vi "ReadDAQConfig.vi"(8 "error in":errorcluster caption="错误输入（无错误）", 11 "产品型号":refnum<vi>) -> (0 "error out":errorcluster caption="错误输出", 3 "DAQConfig":T1={"DIO"=[["ACC", "Dev1/port2/line0", "Dev1/port0/line24"], ["ILL", "Dev1/port2/line1", "Dev1/port0/line25"], ["BACK", "Dev1/port2/line2", "Dev1/port0/line26"], ["BRAKE", "Dev1/port2/line3", "Dev1/port0/line27"], ["PowerON_Vps", "Dev1/port2/line4", "Dev1/port0/line28"], ["PowerON_+B", "Dev1/port2/line5", "Dev1/port0/line29"], ["SW", "Dev1/port2/line6", "Dev1/port0/line30"], ["SW1", "Dev1/port0/line5", "Dev1/port0/line13"], ["SW2", "Dev1/port0/line6", "Dev1/port0/line14"], ["LineOut1", "Dev1/port1/line3", "Dev1/port0/line19"], ["LineOut2", "Dev1/port1/line2", "Dev1/port0/line18"], ["LineOut3", "Dev1/port1/line5", "Dev1/port0/line21"], ["LineOut4", "Dev1/port1/line4", "Dev1/port0/line20"], ["LineOut5", "Dev1/port1/line7", "Dev1/port0/line23"], ["LineOut6", "Dev1/port1/line6", "Dev1/port0/line22"], ["SPK", "Dev1/port2/line7", "Dev1/port0/line31"], ["SPK2", "Dev1/port0/line7", "Dev1/port0/line15"], ["IPOD_DET", "Dev1/port1/line0", "Dev1/port0/line16"], ["RING", "Dev1/port1/line1", "Dev1/port0/line17"], ["PASSButton", "Dev1/port0/line2", "Dev1/port0/line10"], ["FAILButton", "Dev1/port0/line3", "Dev1/port0/line11"], ["DO_IPOD+5V", "Dev1/port0/line4", "Dev1/port0/line12"]], "AO"=[["PowerSimulate", "Dev1/ao0", "Dev1/ao2"], ["AudioSW", "Dev1/ao1", "Dev1/ao3"]], "AI"=[["PowerMonitor", "Dev1/ai5", "Dev1/ai21"], ["FL", "Dev1/ai0", "Dev1/ai16"], ["FR", "Dev1/ai1", "Dev1/ai17"], ["RL", "Dev1/ai2", "Dev1/ai18"], ["RR", "Dev1/ai3", "Dev1/ai19"], ["FLOUT", "Dev1/ai6", "Dev1/ai22"], ["FROUT", "Dev1/ai7", "Dev1/ai23"], ["RLOUT", "Dev1/ai13", "Dev1/ai29"], ["RROUT", "Dev1/ai14", "Dev1/ai30"], ["SUB", "Dev1/ai15", "Dev1/ai31"], ["Current", "Dev1/ai4", "Dev1/ai20"], ["IPOD+5V", "Dev1/ai12", "Dev1/ai28"]]})   [LabVIEW 2013]
uses:
  Controls/DAQConfig.ctl
  <vilib>/Utility/NIReport.llb/NI_report.lvclass
  GlobalValue.vi
  <vilib>/addons/_office/excel.llb/Excel Get Data ([str]).vi
  <vilib>/addons/_office/NI_ReportGenerationToolkit.lvlib
  <vilib>/Utility/NIReport.llb/Excel/NI_Excel.lvclass
panel:
  out "AI":string[][](table)=[["PowerMonitor", "Dev1/ai5", "Dev1/ai21"], ["FL", "Dev1/ai0", "Dev1/ai16"], ["FR", "Dev1/ai1", "Dev1/ai17"], ["RL", "Dev1/ai2", "Dev1/ai18"], ["RR", "Dev1/ai3", "Dev1/ai19"], ["FLOUT", "Dev1/ai6", "Dev1/ai22"], ["FROUT", "Dev1/ai7", "Dev1/ai23"], ["RLOUT", "Dev1/ai13", "Dev1/ai29"], ["RROUT", "Dev1/ai14", "Dev1/ai30"], ["SUB", "Dev1/ai15", "Dev1/ai31"], ["Current", "Dev1/ai4", "Dev1/ai20"], ["IPOD+5V", "Dev1/ai12", "Dev1/ai28"]]
  out "AO":string[][](table)=[["PowerSimulate", "Dev1/ao0", "Dev1/ao2"], ["AudioSW", "Dev1/ao1", "Dev1/ao3"]]
  out "DO":string[][](table)=[["ACC", "Dev1/port2/line0", "Dev1/port0/line24"], ["ILL", "Dev1/port2/line1", "Dev1/port0/line25"], ["BACK", "Dev1/port2/line2", "Dev1/port0/line26"], ["BRAKE", "Dev1/port2/line3", "Dev1/port0/line27"], ["PowerON_Vps", "Dev1/port2/line4", "Dev1/port0/line28"], ["PowerON_+B", "Dev1/port2/line5", "Dev1/port0/line29"], ["SW", "Dev1/port2/line6", "Dev1/port0/line30"], ["SW1", "Dev1/port0/line5", "Dev1/port0/line13"], ["SW2", "Dev1/port0/line6", "Dev1/port0/line14"], ["LineOut1", "Dev1/port1/line3", "Dev1/port0/line19"], ["LineOut2", "Dev1/port1/line2", "Dev1/port0/line18"], ["LineOut3", "Dev1/port1/line5", "Dev1/port0/line21"], ["LineOut4", "Dev1/port1/line4", "Dev1/port0/line20"], ["LineOut5", "Dev1/port1/line7", "Dev1/port0/line23"], ["LineOut6", "Dev1/port1/line6", "Dev1/port0/line22"], ["SPK", "Dev1/port2/line7", "Dev1/port0/line31"], ["SPK2", "Dev1/port0/line7", "Dev1/port0/line15"], ["IPOD_DET", "Dev1/port1/line0", "Dev1/port0/line16"], ["RING", "Dev1/port1/line1", "Dev1/port0/line17"], ["PASSButton", "Dev1/port0/line2", "Dev1/port0/line10"], ["FAILButton", "Dev1/port0/line3", "Dev1/port0/line11"], ["DO_IPOD+5V", "Dev1/port0/line4", "Dev1/port0/line12"]]
  out "ConfigPath":string="D:\\导航\\AVN\\config\\DAQConfig.xls"
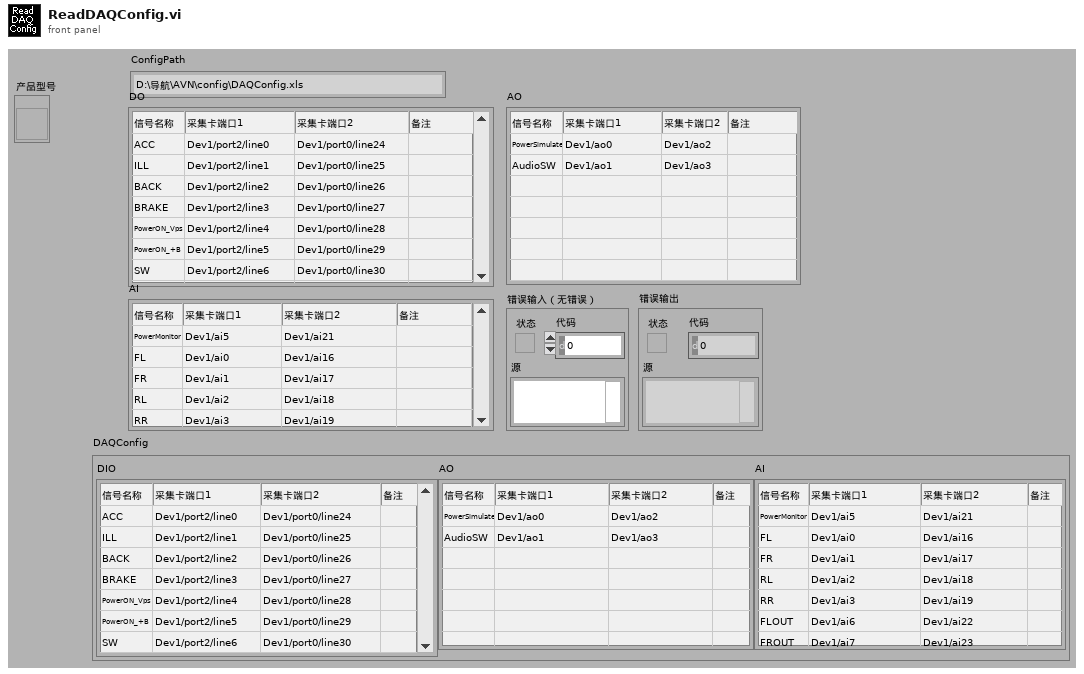
[diagram p1: front panel]
types:
  T1 = typedef "DAQConfig.ctl" = cluster{"DIO":string[][], "AO":string[][], "AI":string[][]}
  T2 = enum16{"maximized", "minimized", "normal", "no change"}
  T3 = enum16{"Standard Report", "HTML", "Word", "Excel"}
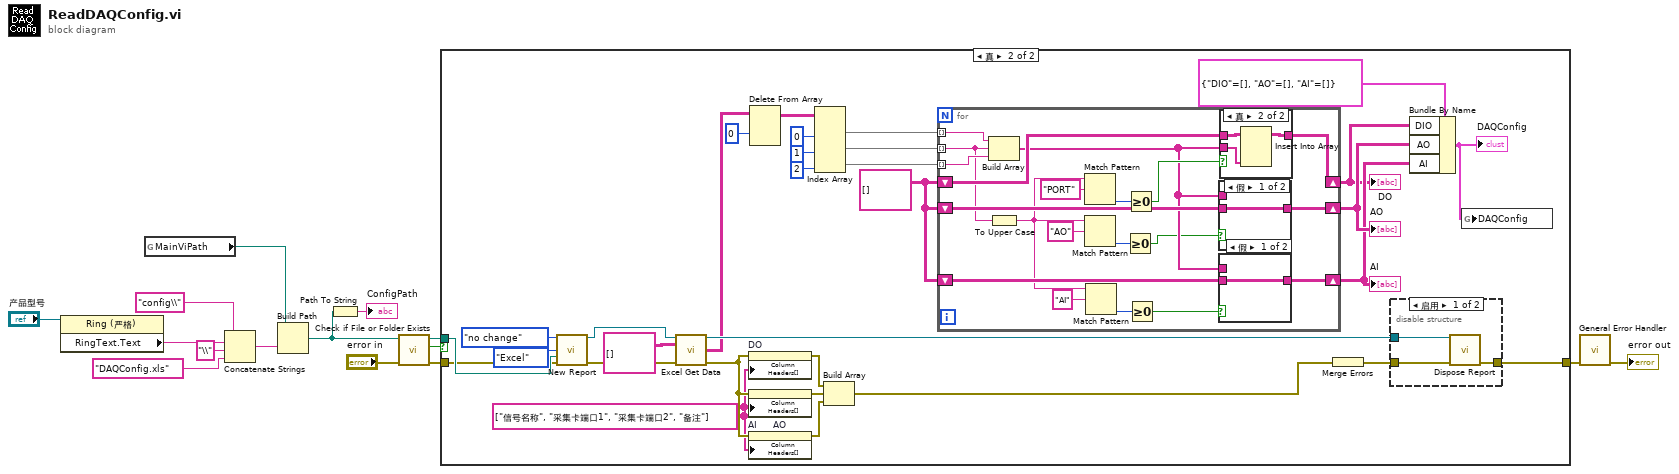
[diagram p0: block diagram]
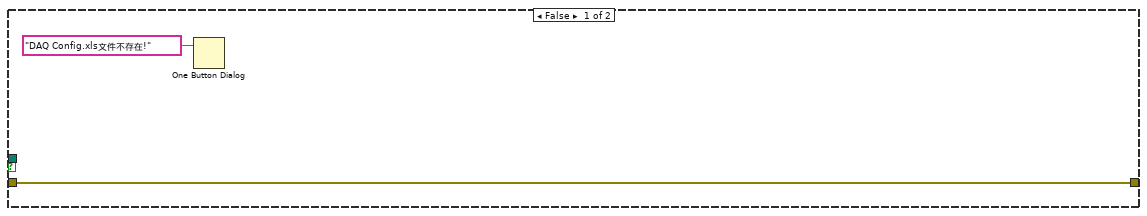
[diagram p2: hidden frame]
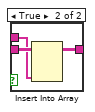
[diagram p4: hidden frame]
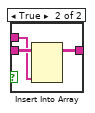
[diagram p6: hidden frame]
diagram:
  n1 = property on="属性节点" class="Ring (严格)"(reference="产品型号") -> ("RingText.Text"=w3:string)  [unwired: 1 in, 2 out]
  n2 = global read "GlobalValue.vi" "MainViPath"() -> (w7:path)
  n3 = Concatenate Strings("config\\" ("连接的字符串"), w3, "\\" ("字符串"), "DAQConfig.xls" ("连接的字符串")) -> (w1:string)
  n4 = Build Path(base path=w7, name or relative path=w1) -> (appended path=w12:path)
  n5 = Path To String(path=w12) -> (string=→"ConfigPath":string)
  n6 = call <vilib>:"Check if File or Folder Exists.vi"("error in (no error)"="error in", "path"=w12) -> ("error out"=w15:errorcluster, "file or folder exists?"=w14:bool, "dup path"=w9:path)  [unwired: 7 out]
  n7 = case shown="真" w14 {
    tunnel: w15 -> [w17 w47]
    tunnel: w9 -> [_ w48]
    tunnel: [w17 w45] -> w13
    frame False {
      n8 = One Button Dialog(message="DAQ Config.xls文件不存在!" ("消息")) -> ()  [unwired: 1 in, 1 out]
    }
    frame True {
      w26 = string[] ["信号名称", "采集卡端口1", "采集卡端口2", "备注"] ("已删除的部分")
      w24 = string[][] [] ("Array")
      n9 = call <vilib>:"New Report.vi"("window state (normal)"=T2."no change", "report type"=T3."Excel", "template (empty)"=w48, "error in (no error)"=w47) -> ("report out"=w40:refnum<class "NI_report.lvclass">, "error out"=w38:errorcluster)  [unwired: 2 in, 8 out]
      n10 = call-poly <vilib>:"Excel Get Data.vi"("report in"=w40, "data type"=string[][] [], "error in (no error)"=w38) -> ("report out"=w46:refnum<class "NI_report.lvclass">, "data"=w37:string[][], "error out"=w27:errorcluster)  [unwired: 10 in]
      n11 = property on="DO" class="Tbl (严格)"(error in=w27, "Column Headers[]"=w26) -> (error out=w22:errorcluster)  [unwired: 1 in, 1 out]
      n12 = property on="AO" class="Tbl (严格)"(error in=w27, "Column Headers[]"=w26) -> (error out=w39:errorcluster)  [unwired: 1 in, 1 out]
      n13 = property on="AI" class="Tbl (严格)"(error in=w27, "Column Headers[]"=w26) -> (error out=w25:errorcluster)  [unwired: 1 in, 1 out]
      n14 = Delete From Array(array=w37, index (row)=0 ("索引 (行)")) -> (array with subset deleted=w35:string[][])  [unwired: 2 in, 1 out]
      n15 = Index Array(array=w35, index (col) #1=0 ("禁用的索引 (列)"), index (col) #2=1 ("索引 (列)"), index (col) #3=2 ("索引 (列)")) -> (element #1=w33:string[], element #2=w21:string[], element #3=w19:string[])  [unwired: 3 in]
      n16 = Build Array(w22, w39, w25) -> (w43:errorcluster[])
      n17 = for {
        shift-right: [w66] -> w23
        shift-left: w24 -> [w65]
        shift-right: [w70] -> w29
        shift-left: w24 -> [w69]
        tunnel: w33 -> [w58] mode=indexing
        shift-right: [w62] -> w28
        shift-left: w24 -> [w63]
        tunnel: w21 -> [w57] mode=indexing
        tunnel: w19 -> [w61] mode=indexing
        n18 = Build Array(w58, w57, w61) -> (w59:string[])
        n19 = To Upper Case(1:w57) -> (0:w60:string)
        n20 = Match Pattern(string=w60, regular expression="PORT") -> (offset past match=w56:i32)  [unwired: 1 in, 3 out]
        n21 = Match Pattern(string=w60, regular expression="AO") -> (offset past match=w55:i32)  [unwired: 1 in, 3 out]
        n22 = Match Pattern(string=w60, regular expression="AI") -> (offset past match=w53:i32)  [unwired: 1 in, 3 out]
        n23 = Greater Or Equal To 0?(x=w55) -> (x >= 0?=w54:bool)
        n24 = Greater Or Equal To 0?(x=w56) -> (x >= 0?=w67:bool)
        n25 = Greater Or Equal To 0?(x=w53) -> (x >= 0?=w52:bool)
        n26 = case shown="假" w54 {
          tunnel: [w80 w82] -> w70
          tunnel: w69 -> [w80 w83]
          tunnel: w59 -> [_ w81]
          frame False {
          }
          frame True {
            n27 = Insert Into Array(array=w83, new element=w81) -> (w82:string[][])  [unwired: 2 in]
          }
        }
        n28 = case shown="假" w52 {
          tunnel: [w72 w74] -> w62
          tunnel: w63 -> [w72 w75]
          tunnel: w59 -> [_ w73]
          frame False {
          }
          frame True {
            n29 = Insert Into Array(array=w75, new element=w73) -> (w74:string[][])  [unwired: 2 in]
          }
        }
        n30 = case shown="真" w67 {
          tunnel: [w76 w78] -> w66
          tunnel: w65 -> [w76 w79]
          tunnel: w59 -> [_ w77]
          frame False {
          }
          frame True {
            n31 = Insert Into Array(array=w79, new element=w77) -> (w78:string[][])  [unwired: 2 in]
          }
        }
      }
      "DO" <- w23
      "AO" <- w29
      "AI" <- w28
      n32 = Merge Errors(w43) -> (w42:errorcluster)
      n33 = disable-structure shown="启用" {
        disable-tunnel: w46 -> [w51 _]
        disable-tunnel: [w50 _] -> w45
        disable-tunnel: w42 -> [w49 _]
        frame Enabled {
          n34 = call-dynamic "Dispose Report.vi"("report in"=w51, "error in (no error)"=w49) -> ("error out"=w50:errorcluster)  [unwired: 3 in, 10 out]
        }
        frame Disabled {
        }
      }
      n35 = Bundle By Name(cluster=T1 {"DIO"=[], "AO"=[], "AI"=[]} ("DAQConfig"), "DIO"=w23, "AO"=w29, "AI"=w28) -> (w18:T1)
      "DAQConfig" <- w18
      n36 = global write "GlobalValue.vi" "DAQConfig"(w18) -> ()
    }
  }
  n37 = call <vilib>:"General Error Handler.vi"("error in (no error)"=w13) -> ("error out"=→"error out":errorcluster)  [unwired: 10 in, 4 out]
